vi "DMCConfiguatorGui.FileRead.vi"(8 "error in (no error)":errorcluster) -> (0 "error out":errorcluster, 2 "ConfigData":T1[](array[typedef]))   [LabVIEW 2016]
uses:
  DMCConfiguatorGui.ConfigData.ctl
  DMCConfiguatorGui.Component.ctl
  DMCConfiguatorGui.Type.ctl
  DMCConfiguatorGui.Var.ctl
  tools/Translator/Translator.Message.ctl
  tools/Translator/Translator.FormatMessage.vi
  Global/ApplicationGlobal.vi
  tools/Translator/Translator.Global.vi
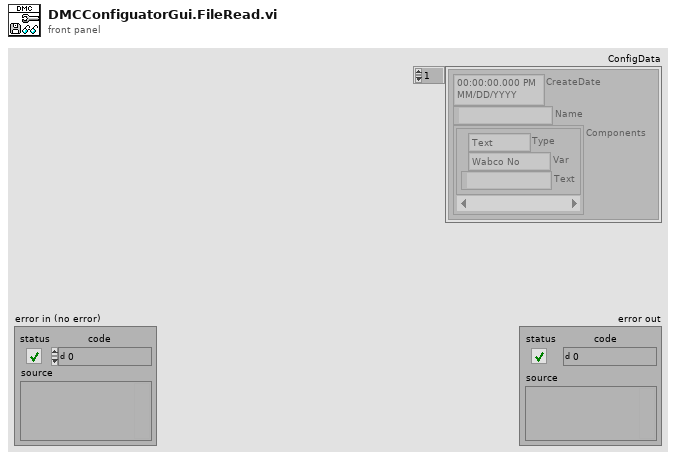
[diagram p1: front panel]
types:
  T1 = typedef "DMCConfiguatorGui.ConfigData.ctl" = cluster{"CreateDate":timestamp, "Name":string, "Components":T2[]}
  T2 = typedef "DMCConfiguatorGui.Component.ctl" = cluster{"Type":T3, "Var":T4, "Text":string}
  T3 = typedef "DMCConfiguatorGui.Type.ctl" = enum8{"Text", "Variable"}
  T4 = typedef "DMCConfiguatorGui.Var.ctl" = enum8{"-", "Wabco No", "Client No", "Serial", "Date"}
  T5 = typedef "Translator.Message.ctl" = enum16{"-", "Event confirmed", "Log out", "Log in", "Shutdown", "Cancel", "Start", "Begin time", "End time", "Duration", "Service Mode", "Ignore Results", "Serial Format", "On", "Off", "OK", "NOK", "NOK %s", "Home", "Work", "Close", "Open", "In progress...", "Missing", "Empty", "Hardware failure", "Initial", "Default", "Total", "Out of range", "Free disk space is below 1GB - contact technician", "Error %d >> %s", "Error %d >> %s >> %s", "Msg %d >> %s", "Laser msg %d %s", "Laser cmd error %s %d", "Laser cmd failed %s", "Laser cmd warning %s", "Laser disconnected", "Laser status %s", "Laser already started", "Laser job unkonwn %s", "Laser job missing %s", "Laser job select failure %s", "Unable to start laser printing (%s)", "Unable to stop laser printing (%s)", "Laser marking aborted", "Laser marking timeout", "Unable to reset Laser Interlock (%s)", "Unable to trigger Laser. Laser not ready (%s)", "Laser job '%s' coordinates not configured", "Starting %s", "Quitting %s", "Configured", "Initializing", "Quitting", "Loading", "Loaded %d results", "Loaded %d events", "Running", "Stopped", "Summary", "Laser", "Do you want to continue?", "Do you want to delete the configuration?", "The configuration is being used by an order. Unable to delete!", "Press confirm button", "Station is not based. Do you want to exit?", "Station requires changeover. Do you want to run the test?", "Test options are not set as default. Do you want to continue?", "Formatting of WabcoNo is disabled. Do you want to continue?", "Product not detected. Do you want to continue?", "Product scan failed. Do you want to continue?", "Calibration", "Log out?", "System", "All", "IDLE", "Translating...%s", "Not found", "Alarm %s", "Run", "Skip", "Abort", "Repeat", "Please wait...", "Database disconnected", "Database disconnected - changeover disabled!", "Login to database successful", "Login to database failed: %d; %s", "Unable to check the product status of reference %d - database disconnected", "Unable to set the product status of reference %d - database disconnected", "Variant file backup %s", "Read variant (%s)", "Result", "Station armed!", "Station requires changeover!", "Select reference number...", "EMERGENCY BUTTON - press Control button", "EMERGENCY DOOR - press Control button", "Resetting Emergency...", "Unable to reset safety circuit - Emergency Button pressed", "Unable to reset safety circuit - Emergency Side Door open", "Station not based", "Station based", "Station not empty", "Station basing...", "No order", "Press Start to begin new order", "Scanning new order", "Order NOK. Correct or scan again", "Order OK. Press Accept", "Order ready", "Revolver incorrect", "Fork incorrect", "Revolver missing", "Revolver empty", "Container missing", "Offline results", "Offline statistics", "Updating statistics %.1f %%", "DMC Configurator", "Door open", "Close the front door", "Press start button", "Done. Open the front door", "Running...", "Running...%.1f %%", "Pause %s", "Pause %s. NOK container missing", "Pause %s. OK container missing", "Pause %s. Revolver empty", "Pause %s. Revolver missing", "Pause %s. Revolver incorrect", "Pause %s. Fork missing", "Pause %s. Fork incorrect", "Pause %s. Too many failures", "Pause %s. Unloading failure", "Pause %s. One slot is not working", "Pause %s. Part order is done. Empty OK container", "Pause %s. Unable to move product to slot", "Pause %s. Unable to move back product pusher", "Pause %s. Unable to lift product", "Pause %s. Unable to move back product lifter", "Pause %s. Unable to move product arm to Work", "Pause %s. Unable to move product arm to NOK", "Pause %s. Unable to move product arm to OK", "Pause %s. Unable to unsuck the NOK product", "Pause %s. Unable to drop the NOK product", "Pause %s. Product OK missing", "Pause %s. Unable to unsuck the OK product", "Pause %s. Unable to drop the OK product", "Stopping...", "File '%s' is missing", "File '%s' is broken", "File '%s' is running", "Log file started (%s)", "Log file ended (%s)", "Log file stopped (%s)", "Log file ignored (%s)", "Log file exported (%s)", "Log file export failed (%s)", "Wrong serial number in log file", "Wrong reference number in log file", "Test steps are missing", "%s = %.3f", "Process param '%s' not found in DB", "Process param '%s' wrong order", "Process param '%s' value %.3f out of limits (%.3f; %.3f)", "Step%d param '%s' not found in DB", "Step%d param '%s' wrong order", "Step%d param '%s' value %.3f out of limits (%.3f; %.3f)", "Step%d EV '%s' not found in DB", "Step%d EV '%s' wrong order", "\"%s\" not found in DB", "\"%s\" wrong order", "\"%s\" value %.3f out of limits (%.3f; %.3f)", "\"%s\" not found in software", "Process init (%s)", "Process started", "Process restarted", "Process run", "Process done", "Process done - remove OK container", "Process aborted", "Process aborted at work", "Process aborted at home", "Process error", "Process error at home", "Process error at work", "Process close", "Process pause", "Process continue", "Process door open", "Process door close", "Process pause at slot %s due to %s", "Select plate from the order to process", "Do you want to start the process?", "Do you want to continue the process?", "There is unfinished order. Do you want to put the new order?", "Product %s %d OK", "Product %s %d NOK", "Unable to unload the slot %s. Product missing in the slot", "Unable to unload the slot %s. Product already in the arm", "Unable to accept the product as OK. Product missing in slot %s", "Unable to accept the product as OK. Product could not drop into the container at slot %s", "Unable to accept the product as NOK. Product could not drop into the container at slot %s", "Scan failed. Error %s", "Scan failed. Scanner disconnected", "Scan failed. Wrong Wabco number %d, limit (%d,%d)", "Scan failed. Wrong serial number %d, limit (%d,%d)", "Scan failed. Wrong date %d, limit (%d,%d)", "Scan failed. Wrong product wabco number %d (expected %d)", "Scan failed. Wrong product serial number %d (expected > 0)", "Scan OK %s", "Scan failed. Unable to determine table position (%s)", "Scan failed. Timeout", "Tune failed. Scanner disconnected", "Tune failed. Timeout", "%s = %d", "%s = %d->%d", "Unable to set %s = %.2f - Air Pressure Inside off", "Unable to set digital output '%s' = %d", "Unable to activate air pressure inside - timeout", "Unable to activate air pressure inside - aborted", "Unable to switch on Air Main Valve - Air Pressure Inlet off", "Unable to switch on Air Main Valve - Door open", "Unable to switch off Air Main Valve - timeout", "Unable to switch off Air Main Valve - aborted", "Unable to rotate Table - timeout", "Unable to rotate Table - aborted", "Unable to rotate Table - Product Move not in Home position", "Unable to rotate Table - Air Pressure Inside off", "Unable to rotate Table - Product Lift A not in Home position", "Unable to rotate Table - Product Lift B not in Home position", "Unable to rotate Table - unlock before movement timeout", "Unable to rotate Table - lock after movement timeout", "Unable to move Table Lock to %s position - timeout", "Unable to move Table Lock to %s position - aborted", "Unable to move Table Lock to %s position - Air Pressure Inside off", "Unable to move Table Lock to %s position - Table not in position", "Unable to move Product Lift A to %s position - timeout", "Unable to move Product Lift B to %s position - timeout", "Unable to move Product Lift A to %s position - aborted", "Unable to move Product Lift B to %s position - aborted", "Unable to move Product Lift A to %s position - Air Pressure Inside off", "Unable to move Product Lift B to %s position - Air Pressure Inside off", "Unable to move Product Lift A to %s position - Table not locked", "Unable to move Product Lift B to %s position - Table not locked", "Unable to move Product Lift A to %s position - Product Arm not in Work position", "Unable to move Product Lift B to %s position - Product Arm not in Work position", "Unable to set Product Suction Gripper %s to %s - timeout", "Unable to set Product Suction Gripper %s to %s - aborted", "Unable to set Product Suction Gripper %s to %s - Air Pressure Inside off", "Unable to set Product Suction Gripper %s to %s - Table slot unkown", "Unable to move Product Arm to %s position - timeout", "Unable to move Product Arm to %s position - aborted", "Unable to move Product Arm to %s position - Air Pressure Inside off", "Unable to move Product Arm to %s position - Product Lift A not in Home position", "Unable to move Product Arm to %s position - Product Lift B not in Home position", "Unable to move Product to %s position - timeout", "Unable to move Product to %s position - aborted", "Unable to move Product to %s position - Air Pressure Inside off", "Unable to move Product to %s position - Table not in position"}
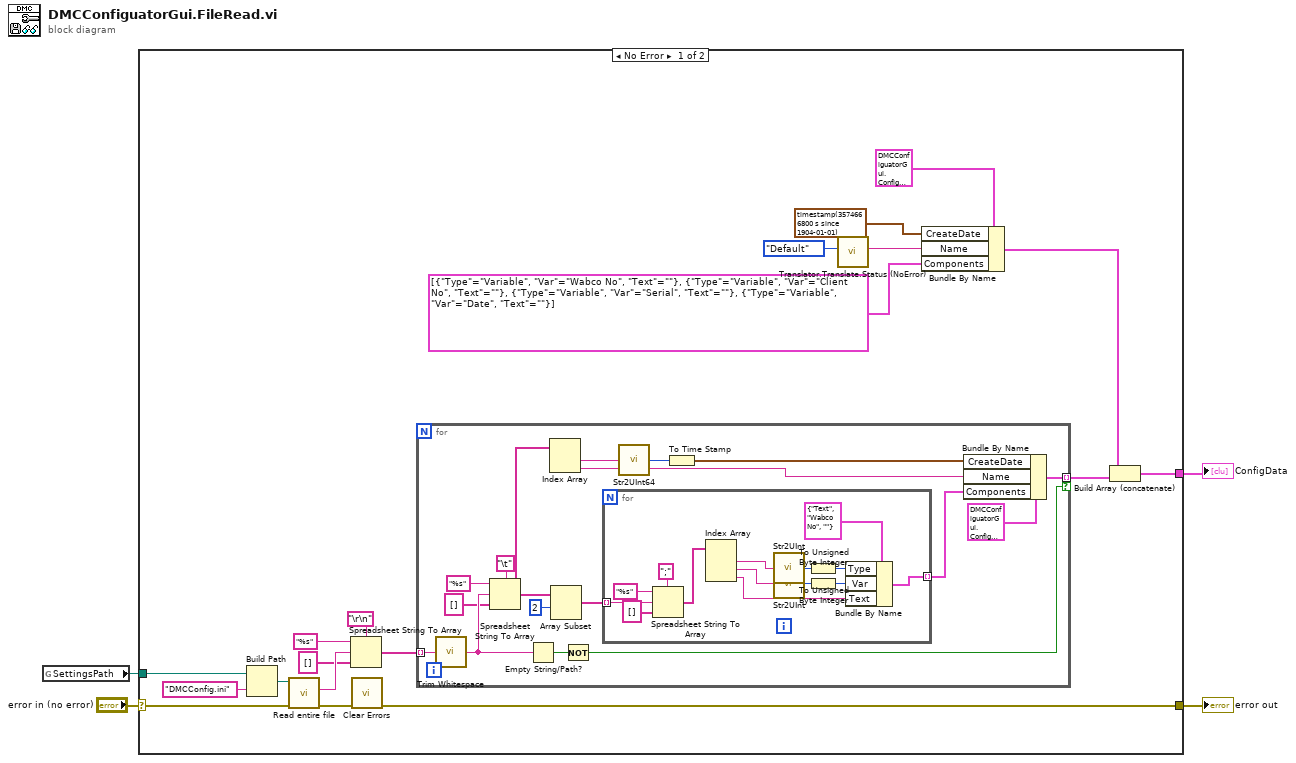
[diagram p0: block diagram]
diagram:
  n1 = global read "ApplicationGlobal.vi" "SettingsPath"() -> (w2:path)
  n2 = case shown="No Error" "error in (no error)" {
    selector: "error in (no error)" -> [w19 w55]
    tunnel: [w18 w55] -> w3
    tunnel: w2 -> [w22 _]
    tunnel: [w7 _] -> w1
    frame No Error {
      n3 = Build Path(base path=w22, name or relative path="DMCConfig.ini" ("format string")) -> (appended path=w20:path)
      n4 = call "Read entire file.vi"("error in"=w19, "file"=w20) -> ("error out"=w23:errorcluster, "contents"=w15:string)  [unwired: 4 in]
      n5 = Spreadsheet String To Array(delimiter (Tab)="\r\n", format string="%s", spreadsheet string=w15, array type (2D Dbl)=string[] []) -> (array=w14:string[])
      n6 = call <vilib>:"Clear Errors.vi"("error in (no error)"=w23) -> ("error out"=w18:errorcluster)  [unwired: 5 in, 1 out]
      n7 = for {
        tunnel: w14 -> [w40] mode=indexing
        tunnel: [w26] -> w12 mode=indexing if=w25
        n8 = call <vilib>:"Trim Whitespace.vi"("string"=w40) -> ("trimmed string"=w38:string)  [unwired: 1 in]
        n9 = Spreadsheet String To Array(delimiter (Tab)="\t", format string="%s", spreadsheet string=w38, array type (2D Dbl)=string[] []) -> (array=w33:string[])
        n10 = Empty String/Path?(string/path=w38) -> (empty?=w39:bool)
        n11 = Index Array(array=w33) -> (element #1=w32:string, element #2=w29:string)  [unwired: 2 in]
        n12 = Array Subset(array=w33, index=2) -> (w34:string[])  [unwired: 1 in]
        n13 = Not(x=w39) -> (.not. x?=w25:bool)
        n14 = for {
          tunnel: w34 -> [w47] mode=indexing
          tunnel: [w41] -> w27 mode=indexing
          n15 = Spreadsheet String To Array(delimiter (Tab)=";", format string="%s", spreadsheet string=w47, array type (2D Dbl)=string[] []) -> (array=w42:string[])
          n16 = Index Array(array=w42) -> (element #1=w45:string, element #2=w44:string, element #3=w43:string)  [unwired: 3 in]
          n17 = call "Str2UInt.vi"("string"=w45) -> ("Numeric"=w54:u32)
          n18 = call "Str2UInt.vi"("string"=w44) -> ("Numeric"=w53:u32)
          n19 = To Unsigned Byte Integer(number=w54) -> (unsigned 8bit integer=w51:u8)
          n20 = To Unsigned Byte Integer(number=w53) -> (unsigned 8bit integer=w50:u8)
          n21 = Bundle By Name(cluster=T2 {"Type"=enum."Text", "Var"=enum."Wabco No", "Text"=""} ("Component"), "Type"=w51, "Var"=w50, "Text"=w43) -> (w41:T2)
        }
        n22 = call "Str2UInt64.vi"("string"=w32) -> ("Numeric"=w31:u64)
        n23 = To Time Stamp(1:w31) -> (0:w28:timestamp)
        n24 = Bundle By Name(cluster=T1 {"CreateDate"=timestamp(0 s since 1904-01-01), "Name"="", "Components"=[]} ("ConfigData"), "CreateDate"=w28, "Name"=w29, "Components"=w27) -> (w26:T1)
      }
      n25 = call "Translator.Translate.Status (NoError).vi"("msg"=Translator.Message."Default") -> ("Translated Msg"=w9:string)  [unwired: 10 in]
      n26 = Bundle By Name(cluster=T1 {"CreateDate"=timestamp(0 s since 1904-01-01), "Name"="", "Components"=[]} ("ConfigData"), "CreateDate"=timestamp(3574666800 s since 1904-01-01) ("CreateDate 2"), "Name"=w9, "Components"=T2[] [{"Type"=enum."Variable", "Var"=enum."Wabco No", "Text"=""}, {"Type"=enum."Variable", "Var"=enum."Client No", "Text"=""}, {"Type"=enum."Variable", "Var"=enum."Serial", "Text"=""}, {"Type"=enum."Variable", "Var"=enum."Date", "Text"=""}]) -> (w6:T1)
      n27 = Build Array (concatenate)(w6, w12) -> (w7:T1[])
    }
    frame Error {
    }
  }
  "error out" <- w3
  "ConfigData" <- w1
